vi "Get Local Personalities.vi"(8 "error in (no error)":errorcluster) -> (0 "error out":errorcluster, 3 "Personalities":string[](array[string]))   [LabVIEW 2018, in "Personalities Tool.lvlib"]
uses:
  Personalities Tool.lvlib
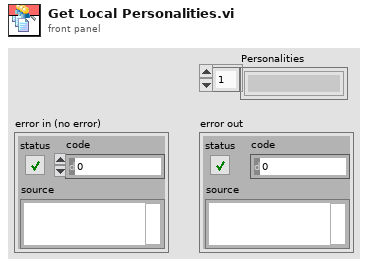
[diagram p1: front panel]
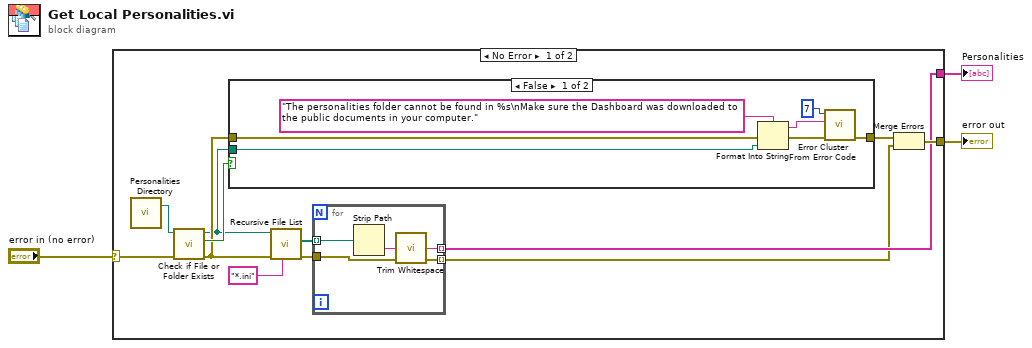
[diagram p0: block diagram]
diagram:
  n1 = case shown="No Error" "error in (no error)" {
    selector: "error in (no error)" -> [w9 w28]
    tunnel: [w15 w28] -> w3
    tunnel: [w14 _] -> w2
    frame No Error {
      n2 = call "Personalities Directory.vi"() -> ("appended path"=w7:path)  [unwired: 3 in]
      n3 = call <vilib>:"Check if File or Folder Exists.vi"("error in (no error)"=w9, "path"=w7) -> ("error out"=w6:errorcluster, "file or folder exists?"=w8:bool, "dup path"=w4:path)  [unwired: 7 in]
      n4 = case shown="False" w8 {
        tunnel: w6 -> [w22 w23]
        tunnel: [w21 w23] -> w5
        tunnel: w4 -> [w16 _]
        frame False {
          n5 = Format Into String(format string="The personalities folder cannot be found in %s\nMake sure the Dashboard was downloaded to the public documents in your computer." ("error message (\"\")"), error in=w22, w16) -> (resulting string=w18:string, error out=w19:errorcluster)  [unwired: 1 in]
          n6 = call <vilib>:"Error Cluster From Error Code.vi"("error in (no error)"=w19, "error message (\"\")"=w18, "error code (0)"=7) -> ("error out"=w21:errorcluster)  [unwired: 6 in]
        }
        frame True {
        }
      }
      n7 = call <vilib>:"Recursive File List.vi"("pattern"="*.ini", "error in (no error)"=w6, "Folder Path"=w4) -> ("error out"=w12:errorcluster, "All Files in Dir"=w11:path[])  [unwired: 4 in, 3 out]
      n8 = for {
        tunnel: w11 -> [w26] mode=indexing
        tunnel: [w24] -> w14 mode=indexing
        tunnel: w12 -> [w27]
        tunnel: [w27] -> w13 mode=indexing
        n9 = Strip Path(path=w26) -> (name=w25:string)  [unwired: 1 out]
        n10 = call <vilib>:"Trim Whitespace.vi"("string"=w25) -> ("trimmed string"=w24:string)  [unwired: 1 in]
      }
      n11 = Merge Errors(w5, w13) -> (w15:errorcluster)
    }
    frame Error {
    }
  }
  "error out" <- w3
  "Personalities" <- w2
